vi "UpdateDAQLinescanStatus.vi"(0 "error in (no error)":errorcluster, 1 "Panel":refnum<vi>) -> ()   [LabVIEW 2009]
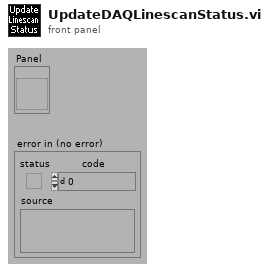
[diagram p1: front panel]
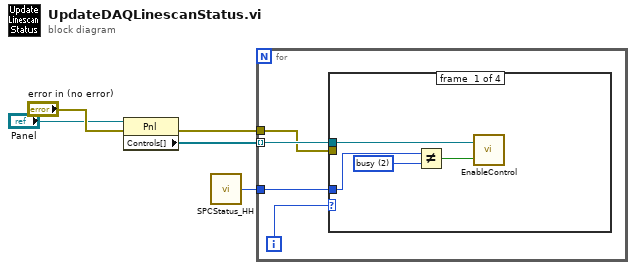
[diagram p0: block diagram]
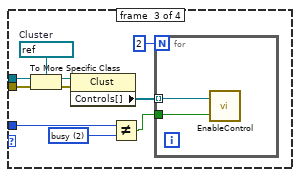
[diagram p3: hidden frame]
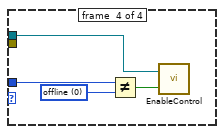
[diagram p4: hidden frame]
diagram:
  n1 = property class="Pnl"(reference="Panel", error in="error in (no error)") -> (error out=w5:errorcluster, "Controls[]"=w2:refnum<vi>[])  [unwired: 1 out]
  n2 = call "SPCStatus_HH.vi"() -> ("Status (output)"=w3:enum16{"offline", "online", "busy"})  [unwired: 2 in]
  n3 = for {
    tunnel: w2 -> [w8] mode=indexing
    tunnel: w3 -> [w6]
    tunnel: w5 -> [w7]
    i -> [w9]
    n4 = case shown="10, 11" w9 {
      tunnel: w8 -> [w13 _ w23 w26]
      tunnel: w7 -> [_ _ w19 _]
      tunnel: w6 -> [w10 _ w14 w28]
      frame #0 {
        w12 = u16 2 items=["offline", "online", "busy"] ("Status (input)")
        n5 = Not Equal?(x=w10, y=w12) -> (x != y?=w11:bool)
        n6 = call "EnableControl.vi"("Enable"=w11, "Reference"=w13) -> ()
      }
      frame #1 {
      }
      frame #2 {
        w16 = u16 2 items=["offline", "online", "busy"] ("Status (input)")
        w22 = refnum<vi> refnum  # Cluster
        n7 = To More Specific Class(target class=w22, reference=w23, error in=w19) -> (specific class reference=w20:refnum<vi>, error out=w21:errorcluster)
        n8 = property class="Clust"(reference=w20, error in=w21) -> ("Controls[]"=w18:refnum<vi>[])  [unwired: 2 out]
        n9 = Not Equal?(x=w14, y=w16) -> (x != y?=w15:bool)
        n10 = for {
          N: 2 -> [_]
          tunnel: w18 -> [w25] mode=indexing
          tunnel: w15 -> [w24]
          n11 = call "EnableControl.vi"("Enable"=w24, "Reference"=w25) -> ()
        }
      }
      frame #3 {
        w29 = u16 0 items=["offline", "online", "busy"] ("Status (input)")
        n12 = Not Equal?(x=w28, y=w29) -> (x != y?=w27:bool)
        n13 = call "EnableControl.vi"("Enable"=w27, "Reference"=w26) -> ()
      }
    }
  }
